vi "ref_gen_proc.vi"(2 "error in (no error)":errorcluster, 3 "B":T1, 4 "A":T1, 5 "wd":dbl) -> (0 "error out":errorcluster, 1 "xkp1":T1)   [LabVIEW 2021]
uses:
  <vilib>/Analysis/Matrix/Datatypes/RealMatrix.ctl
  <vilib>/Analysis/Matrix/NI_Matrix.lvlib
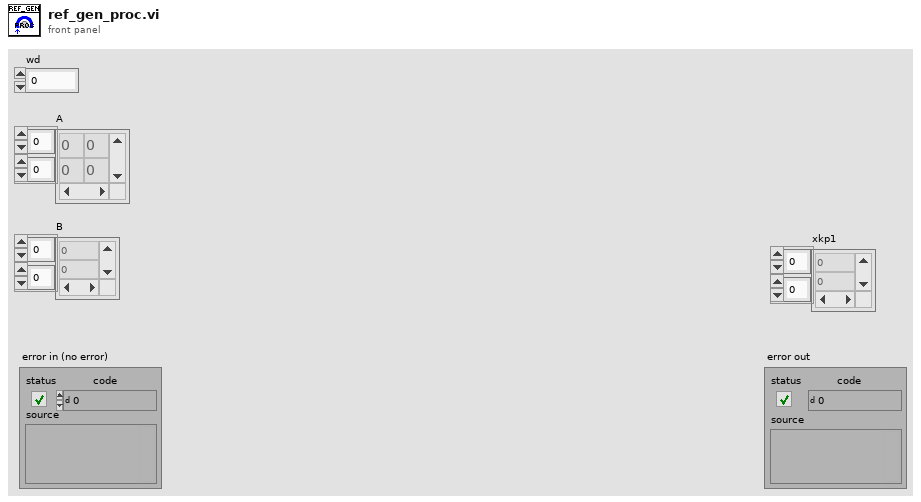
[diagram p1: front panel]
types:
  T1 = typedef "NI_Matrix.lvlib/RealMatrix.ctl" = dbl[][]
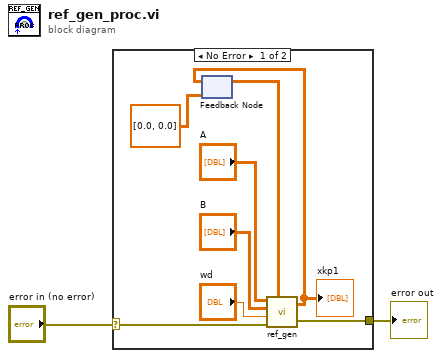
[diagram p0: block diagram]
diagram:
  n1 = case shown="No Error" "error in (no error)" {
    selector: "error in (no error)" -> [w7 w11]
    tunnel: [w6 w11] -> w1
    frame No Error {
      n2 = feedback #1(T1 [[0.0], [0.0]] ("xkp1")) -> (w9:T1)
      n3 = call "ref_gen.vi"("xk"=w9, "error in (no error)"=w7, "wd"="wd", "B"="B", "A"="A") -> ("error out"=w6:errorcluster, "xkp1"=w10:T1)  [unwired: 1 in]
      "xkp1" <- w10
      n4 = feedback-in #1(w10) -> ()
    }
    frame Error {
    }
  }
  "error out" <- w1
